vi "Write_func.vi"(8 "error in (no error)":errorcluster, 10 "cmd":string, 11 "Data Cluster in":T1) -> (0 "error out":errorcluster, 2 "Status":bool, 3 "Data Cluster out":T1)   [LabVIEW 2017, in "FingerPrintMânager.lvlib"]
uses:
  Module Data--cluster.ctl
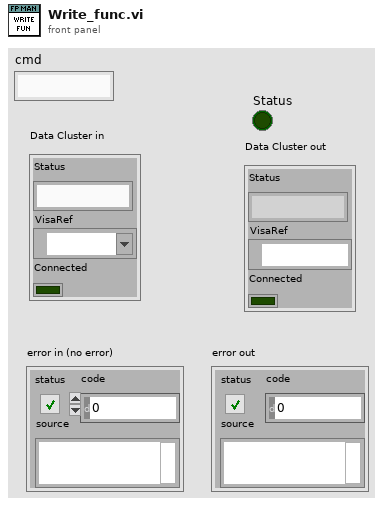
[diagram p1: front panel]
types:
  T1 = typedef "FingerPrintMânager.lvlib/Module Data--cluster.ctl" = cluster{"Status":string, "VisaRef":refnum<visa-resource-name>, "Connected":bool}
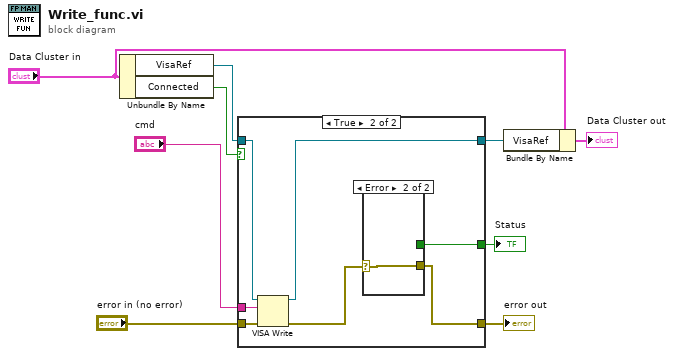
[diagram p0: block diagram]
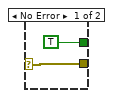
[diagram p3: hidden frame]
diagram:
  n1 = Unbundle By Name("Data Cluster in") -> ("VisaRef"=w4:refnum<visa-resource-name>, "Connected"=w3:bool)
  n2 = case shown="True" w3 {
    tunnel: "error in (no error)" -> [w11 w16]
    tunnel: [w11 w14] -> w7
    tunnel: [w10 w17] -> w9
    tunnel: w4 -> [w10 w18]
    tunnel: "cmd" -> [_ w15]
    tunnel: [_ w12] -> w1
    frame False {
    }
    frame True {
      n3 = VISA Write(VISA resource name=w18, write buffer=w15, error in (no error)=w16) -> (VISA resource name out=w17:refnum<visa-resource-name>, error out=w13:errorcluster)  [unwired: 1 out]
      n4 = case shown="Error" w13 {
        selector: w13 -> [w20 w21]
        tunnel: [w20 w21] -> w14
        tunnel: [TRUE _] -> w12
        frame No Error {
        }
        frame Error {
        }
      }
    }
  }
  "error out" <- w7
  "Status" <- w1
  n5 = Bundle By Name(cluster="Data Cluster in", "VisaRef"=w9) -> (→"Data Cluster out":T1)
